vi "Peregrine_set_hires.vi"(0 "Handle in":refnum<visa-resource-name>, 2 "Address":u8, 11 "error":errorcluster) -> (4 "Handle out":refnum<visa-resource-name>, 6 "Key response":u32, 8 "Value response":i32, 15 "error out":errorcluster)   [LabVIEW 2019]
panel:
  out "Command":i32
  out "Address response":u8
  # "Inputs"
  # "Response message"
  # "Output"
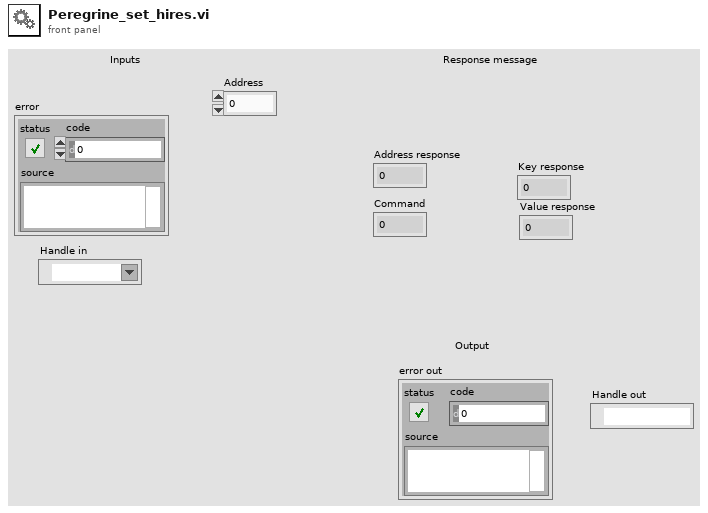
[diagram p1: front panel]
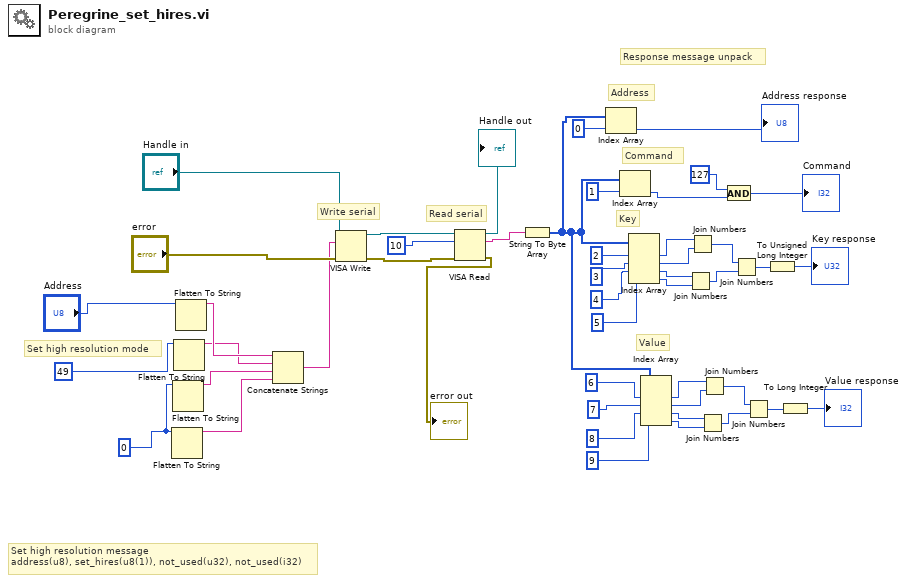
[diagram p0: block diagram]
diagram:
  w1 = 0
  # "Value"
  # "Response message unpack"
  # "Set high resolution mode"
  # "Command"
  # "Address"
  # "Key"
  # "Read serial"
  # "Write serial"
  # "Set high resolution message\naddress(u8), set_hires(u8(1)), not_used(u32), not_used(i32)"
  n1 = Flatten To String(anything=w1) -> (data string=w20:string)  [unwired: 3 in, 2 out]
  n2 = Flatten To String(anything=w1) -> (data string=w21:string)  [unwired: 3 in, 2 out]
  n3 = Flatten To String(anything=u8 49) -> (data string=w22:string)  [unwired: 3 in, 2 out]
  n4 = Flatten To String(anything="Address") -> (data string=w24:string)  [unwired: 3 in, 2 out]
  n5 = Concatenate Strings(w24, w22, w21, w20) -> (w19:string)
  n6 = VISA Write(VISA resource name="Handle in", write buffer=w19, error in (no error)="error") -> (VISA resource name out=w47:refnum<visa-resource-name>, error out=w26:errorcluster)  [unwired: 1 out]
  n7 = VISA Read(VISA resource name=w47, byte count=10, error in (no error)=w26) -> (VISA resource name out=→"Handle out":refnum<visa-resource-name>, read buffer=w45:string, error out=→"error out":errorcluster)  [unwired: 1 out]
  n8 = String To Byte Array(string=w45) -> (unsigned byte array=w11:u8[])
  n9 = Index Array(array=w11, index=0) -> (element=→"Address response":u8)
  n10 = Index Array(array=w11, index=1) -> (element=w3:u8)
  n11 = Index Array(array=w11, index #1=2, index #2=3, index #3=4, index #4=5) -> (element #1=w38:u8, element #2=w37:u8, element #3=w36:u8, element #4=w35:u8)
  n12 = Index Array(array=w11, index #1=6, index #2=7, index #3=8, index #4=9) -> (element #1=w18:u8, element #2=w17:u8, element #3=w16:u8, element #4=w15:u8)
  n13 = Join Numbers(hi=w36, lo=w35) -> ((hi.lo)=w34:u16)
  n14 = Join Numbers(hi=w38, lo=w37) -> ((hi.lo)=w33:u16)
  n15 = Join Numbers(hi=w16, lo=w15) -> ((hi.lo)=w14:u16)
  n16 = Join Numbers(hi=w18, lo=w17) -> ((hi.lo)=w13:u16)
  n17 = And(x=127, y=w3) -> (x .and. y?=→"Command":i32)
  n18 = Join Numbers(hi=w33, lo=w34) -> ((hi.lo)=w6:u32)
  n19 = Join Numbers(hi=w13, lo=w14) -> ((hi.lo)=w7:u32)
  n20 = To Unsigned Long Integer(number=w6) -> (unsigned 32bit integer=→"Key response":u32)
  n21 = To Long Integer(number=w7) -> (32bit integer=→"Value response":i32)
